vi "FlatToRichnixnet_grpc_ReadStateValue.vi"(5 "OutputClusterType":T1, 11 "InputCluster":T2) -> (3 "OutputCluster":T1)   [LabVIEW 2025, in "grpc-xnet_client.lvlib"]
uses:
  grpc-xnet_client.lvlib
  nixnet_grpc_ReadStateValue_Flat.ctl
  nixnet_grpc_CanCommResponse_Flat.ctl
  nixnet_grpc_CanCommState.ctl
  nixnet_grpc_CanLastErr.ctl
  nixnet_grpc_FlexRayCommResponse_Flat.ctl
  nixnet_grpc_FlexRayPocState.ctl
  nixnet_grpc_FlexRayStats_Flat.ctl
  nixnet_grpc_LinCommResponse_Flat.ctl
  nixnet_grpc_LinCommState.ctl
  nixnet_grpc_SessionInfoResponse_Flat.ctl
  nixnet_grpc_SessionInfoState.ctl
  nixnet_grpc_J1939CommState_Flat.ctl
  nixnet_grpc_TimeLocalNetwork_Flat.ctl
  nixnet_grpc_ReadStateValue.ctl
  nixnet_grpc_ReadStateValue_value/nixnet_grpc_ReadStateValue_value.lvclass
  nixnet_grpc_ReadStateValue_value/nixnet_grpc_ReadStateValue_value.lvclass/nixnet_grpc_ReadStateValue_value.ctl
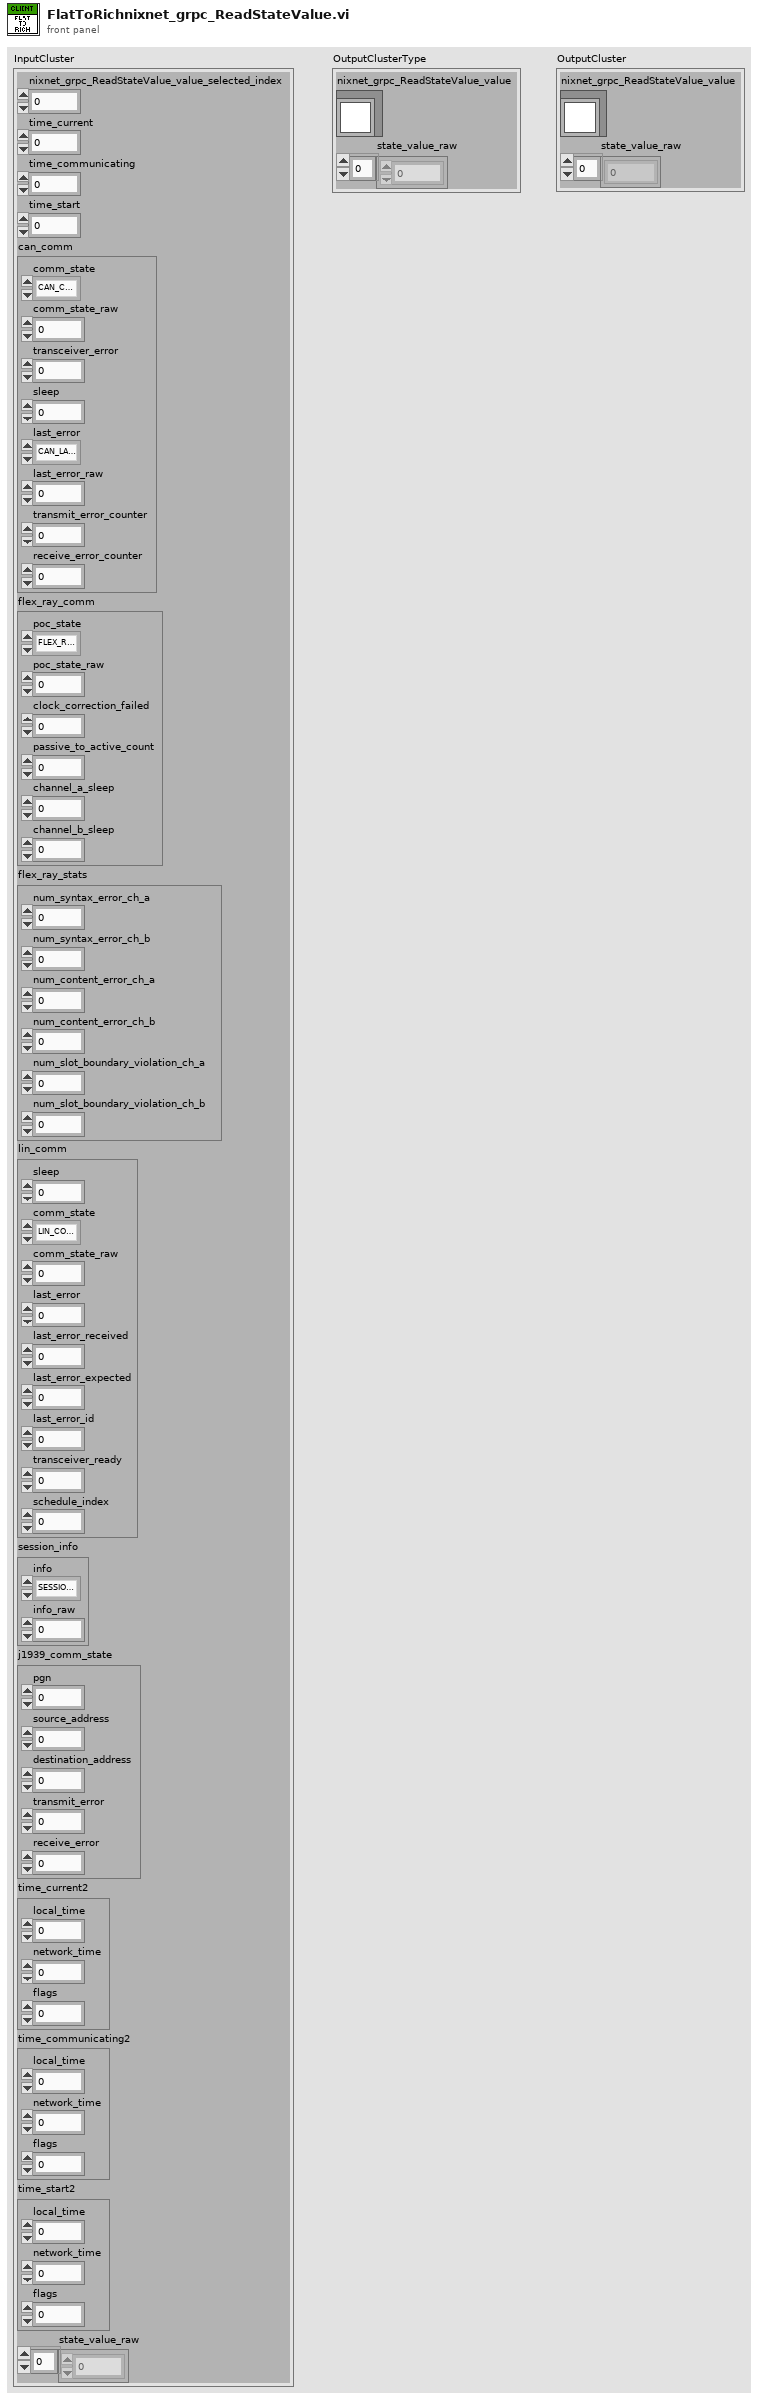
[diagram p1: front panel]
types:
  T1 = typedef "grpc-xnet_client.lvlib/nixnet_grpc_ReadStateValue.ctl" = cluster{"nixnet_grpc_ReadStateValue_value":refnum<class "nixnet_grpc_ReadStateValue_value.lvclass">, "state_value_raw":u8[]}
  T2 = typedef "grpc-xnet_client.lvlib/nixnet_grpc_ReadStateValue_Flat.ctl" = cluster{"nixnet_grpc_ReadStateValue_value_selected_index":i32, "time_current":u64, "time_communicating":u64, "time_start":u64, "can_comm":T3, "flex_ray_comm":T6, "flex_ray_stats":T8, "lin_comm":T9, "session_info":T11, "j1939_comm_state":T13, "time_current2":T14, "time_communicating2":T14, "time_start2":T14, "state_value_raw":u8[]}
  T3 = typedef "grpc-xnet_client.lvlib/nixnet_grpc_CanCommResponse_Flat.ctl" = cluster{"comm_state":T4, "comm_state_raw":u32, "transceiver_error":u32, "sleep":u32, "last_error":T5, "last_error_raw":u32, "transmit_error_counter":u32, "receive_error_counter":u32}
  T4 = typedef "grpc-xnet_client.lvlib/nixnet_grpc_CanCommState.ctl" = enum32{"CAN_COMM_STATE_ERROR_ACTIVE", "CAN_COMM_STATE_ERROR_PASSIVE", "CAN_COMM_STATE_BUS_OFF", "CAN_COMM_STATE_INIT"}
  T5 = typedef "grpc-xnet_client.lvlib/nixnet_grpc_CanLastErr.ctl" = enum32{"CAN_LAST_ERR_NONE", "CAN_LAST_ERR_STUFF", "CAN_LAST_ERR_FORM", "CAN_LAST_ERR_ACK", "CAN_LAST_ERR_BIT_1", "CAN_LAST_ERR_BIT_0", "CAN_LAST_ERR_CRC"}
  T6 = typedef "grpc-xnet_client.lvlib/nixnet_grpc_FlexRayCommResponse_Flat.ctl" = cluster{"poc_state":T7, "poc_state_raw":u32, "clock_correction_failed":u32, "passive_to_active_count":u32, "channel_a_sleep":u32, "channel_b_sleep":u32}
  T7 = typedef "grpc-xnet_client.lvlib/nixnet_grpc_FlexRayPocState.ctl" = enum32{"FLEX_RAY_POC_STATE_DEFAULT_CONFIG", "FLEX_RAY_POC_STATE_READY", "FLEX_RAY_POC_STATE_NORMAL_ACTIVE", "FLEX_RAY_POC_STATE_NORMAL_PASSIVE", "FLEX_RAY_POC_STATE_HALT", "FLEX_RAY_POC_STATE_MONITOR", "FLEX_RAY_POC_STATE_CONFIG"}
  T8 = typedef "grpc-xnet_client.lvlib/nixnet_grpc_FlexRayStats_Flat.ctl" = cluster{"num_syntax_error_ch_a":u32, "num_syntax_error_ch_b":u32, "num_content_error_ch_a":u32, "num_content_error_ch_b":u32, "num_slot_boundary_violation_ch_a":u32, "num_slot_boundary_violation_ch_b":u32}
  T9 = typedef "grpc-xnet_client.lvlib/nixnet_grpc_LinCommResponse_Flat.ctl" = cluster{"sleep":u32, "comm_state":T10, "comm_state_raw":u32, "last_error":u32, "last_error_received":u32, "last_error_expected":u32, "last_error_id":u32, "transceiver_ready":u32, "schedule_index":u32}
  T10 = typedef "grpc-xnet_client.lvlib/nixnet_grpc_LinCommState.ctl" = enum32{"LIN_COMM_STATE_IDLE", "LIN_COMM_STATE_ACTIVE", "LIN_COMM_STATE_INACTIVE"}
  T11 = typedef "grpc-xnet_client.lvlib/nixnet_grpc_SessionInfoResponse_Flat.ctl" = cluster{"info":T12, "info_raw":u32}
  T12 = typedef "grpc-xnet_client.lvlib/nixnet_grpc_SessionInfoState.ctl" = enum32{"SESSION_INFO_STATE_STOPPED", "SESSION_INFO_STATE_STARTED", "SESSION_INFO_STATE_MIX"}
  T13 = typedef "grpc-xnet_client.lvlib/nixnet_grpc_J1939CommState_Flat.ctl" = cluster{"pgn":u32, "source_address":u32, "destination_address":u32, "transmit_error":u32, "receive_error":u32}
  T14 = typedef "grpc-xnet_client.lvlib/nixnet_grpc_TimeLocalNetwork_Flat.ctl" = cluster{"local_time":u64, "network_time":u64, "flags":u32}
  T15 = typedef "grpc-xnet_client.lvlib/nixnet_grpc_CanCommResponse.ctl" = cluster{"comm_state":T4, "comm_state_raw":u32, "transceiver_error":u32, "sleep":u32, "last_error":T5, "last_error_raw":u32, "transmit_error_counter":u32, "receive_error_counter":u32}
  T16 = typedef "grpc-xnet_client.lvlib/nixnet_grpc_FlexRayCommResponse.ctl" = cluster{"poc_state":T7, "poc_state_raw":u32, "clock_correction_failed":u32, "passive_to_active_count":u32, "channel_a_sleep":u32, "channel_b_sleep":u32}
  T17 = typedef "grpc-xnet_client.lvlib/nixnet_grpc_FlexRayStats.ctl" = cluster{"num_syntax_error_ch_a":u32, "num_syntax_error_ch_b":u32, "num_content_error_ch_a":u32, "num_content_error_ch_b":u32, "num_slot_boundary_violation_ch_a":u32, "num_slot_boundary_violation_ch_b":u32}
  T18 = typedef "grpc-xnet_client.lvlib/nixnet_grpc_LinCommResponse.ctl" = cluster{"sleep":u32, "comm_state":T10, "comm_state_raw":u32, "last_error":u32, "last_error_received":u32, "last_error_expected":u32, "last_error_id":u32, "transceiver_ready":u32, "schedule_index":u32}
  T19 = typedef "grpc-xnet_client.lvlib/nixnet_grpc_SessionInfoResponse.ctl" = cluster{"info":T12, "info_raw":u32}
  T20 = typedef "grpc-xnet_client.lvlib/nixnet_grpc_J1939CommState.ctl" = cluster{"pgn":u32, "source_address":u32, "destination_address":u32, "transmit_error":u32, "receive_error":u32}
  T21 = typedef "grpc-xnet_client.lvlib/nixnet_grpc_TimeLocalNetwork.ctl" = cluster{"local_time":u64, "network_time":u64, "flags":u32}
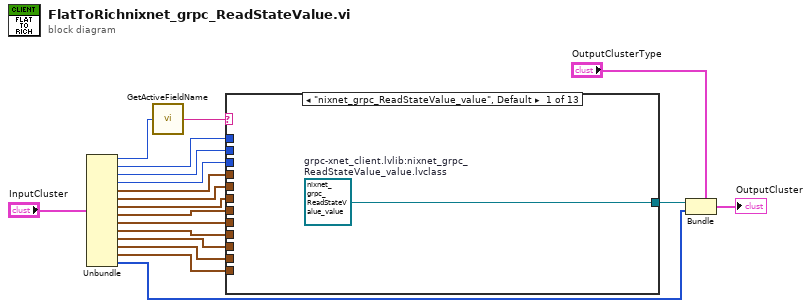
[diagram p0: block diagram]
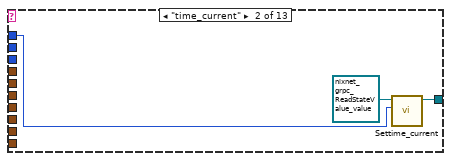
[diagram p2: hidden frame]
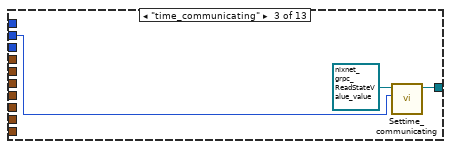
[diagram p3: hidden frame]
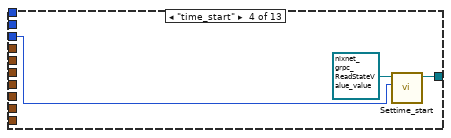
[diagram p4: hidden frame]
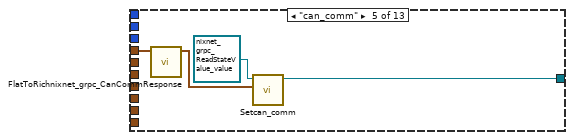
[diagram p5: hidden frame]
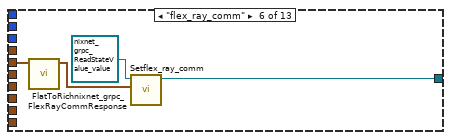
[diagram p6: hidden frame]
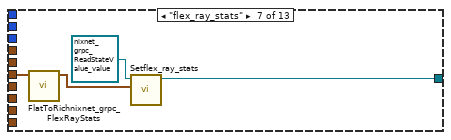
[diagram p7: hidden frame]
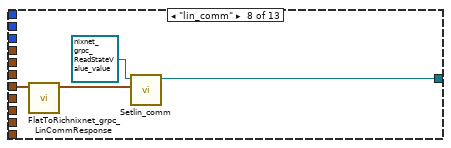
[diagram p8: hidden frame]
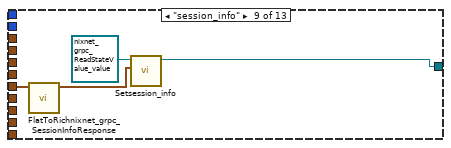
[diagram p9: hidden frame]
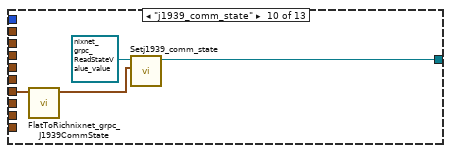
[diagram p10: hidden frame]
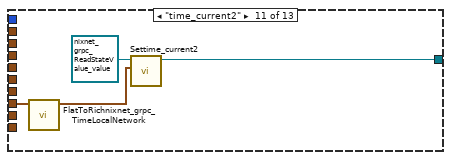
[diagram p11: hidden frame]
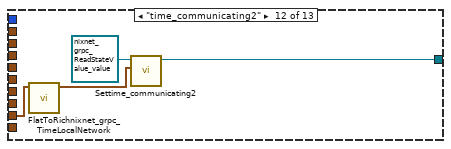
[diagram p12: hidden frame]
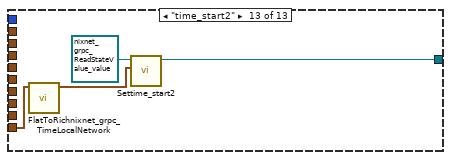
[diagram p13: hidden frame]
diagram:
  n1 = Unbundle "Unbundle"("InputCluster") -> ("nixnet_grpc_ReadStateValue_value_selected_index"=w16:i32, "time_current"=w13:u64, "time_communicating"=w12:u64, "time_start"=w11:u64, "can_comm"=w10:T3, "flex_ray_comm"=w9:T6, "flex_ray_stats"=w8:T8, "lin_comm"=w7:T9, "session_info"=w6:T11, "j1939_comm_state"=w5:T13, "time_current2"=w4:T14, "time_communicating2"=w3:T14, "time_start2"=w2:T14, "state_value_raw"=w1:u8[])
  n2 = call "GetActiveFieldName.vi"("protobuf index"=w16) -> ("oneof field name"=w15:string)
  n3 = case "nixnet_grpc_ReadStateValue_value" shown="\"nixnet_grpc_ReadStateValue_value\", Default" w15 {
    tunnel: [w20 w22 w25 w28 w31 w35 w39 w43 w47 w51 w55 w59 w63] -> w14
    tunnel: w13 -> [_ w23 _ _ _ _ _ _ _ _ _ _ _]
    tunnel: w12 -> [_ _ w26 _ _ _ _ _ _ _ _ _ _]
    tunnel: w11 -> [_ _ _ w29 _ _ _ _ _ _ _ _ _]
    tunnel: w10 -> [_ _ _ _ w33 _ _ _ _ _ _ _ _]
    tunnel: w9 -> [_ _ _ _ _ w37 _ _ _ _ _ _ _]
    tunnel: w8 -> [_ _ _ _ _ _ w41 _ _ _ _ _ _]
    tunnel: w7 -> [_ _ _ _ _ _ _ w45 _ _ _ _ _]
    tunnel: w6 -> [_ _ _ _ _ _ _ _ w49 _ _ _ _]
    tunnel: w5 -> [_ _ _ _ _ _ _ _ _ w53 _ _ _]
    tunnel: w4 -> [_ _ _ _ _ _ _ _ _ _ w57 _ _]
    tunnel: w3 -> [_ _ _ _ _ _ _ _ _ _ _ w61 _]
    tunnel: w2 -> [_ _ _ _ _ _ _ _ _ _ _ _ w65]
    frame "nixnet_grpc_ReadStateValue_value", Default {
      w20 = refnum<class "nixnet_grpc_ReadStateValue_value.lvclass"> refnum  # grpc-xnet_client.lvlib:nixnet_grpc_ReadStateValue_value.lvclass
    }
    frame "time_current" {
      n4 = call "Settime_current.vi"("Set_Val"=w23, "OneOfTemplate in"=refnum<class "nixnet_grpc_ReadStateValue_value.lvclass"> refnum) -> ("OneOfTemplate out"=w22:refnum<class "nixnet_grpc_ReadStateValue_value.lvclass">)  [unwired: 8 in, 1 out]
    }
    frame "time_communicating" {
      n5 = call "Settime_communicating.vi"("Set_Val"=w26, "OneOfTemplate in"=refnum<class "nixnet_grpc_ReadStateValue_value.lvclass"> refnum) -> ("OneOfTemplate out"=w25:refnum<class "nixnet_grpc_ReadStateValue_value.lvclass">)  [unwired: 8 in, 1 out]
    }
    frame "time_start" {
      n6 = call "Settime_start.vi"("Set_Val"=w29, "OneOfTemplate in"=refnum<class "nixnet_grpc_ReadStateValue_value.lvclass"> refnum) -> ("OneOfTemplate out"=w28:refnum<class "nixnet_grpc_ReadStateValue_value.lvclass">)  [unwired: 8 in, 1 out]
    }
    frame "can_comm" {
      n7 = call "FlatToRichnixnet_grpc_CanCommResponse.vi"("InputCluster"=w33) -> ("OutputCluster"=w32:T15)  [unwired: 10 in]
      n8 = call "Setcan_comm.vi"("Set_Val"=w32, "OneOfTemplate in"=refnum<class "nixnet_grpc_ReadStateValue_value.lvclass"> refnum) -> ("OneOfTemplate out"=w31:refnum<class "nixnet_grpc_ReadStateValue_value.lvclass">)  [unwired: 8 in, 1 out]
    }
    frame "flex_ray_comm" {
      n9 = call "FlatToRichnixnet_grpc_FlexRayCommResponse.vi"("InputCluster"=w37) -> ("OutputCluster"=w36:T16)  [unwired: 10 in]
      n10 = call "Setflex_ray_comm.vi"("Set_Val"=w36, "OneOfTemplate in"=refnum<class "nixnet_grpc_ReadStateValue_value.lvclass"> refnum) -> ("OneOfTemplate out"=w35:refnum<class "nixnet_grpc_ReadStateValue_value.lvclass">)  [unwired: 8 in, 1 out]
    }
    frame "flex_ray_stats" {
      n11 = call "FlatToRichnixnet_grpc_FlexRayStats.vi"("InputCluster"=w41) -> ("OutputCluster"=w40:T17)  [unwired: 10 in]
      n12 = call "Setflex_ray_stats.vi"("Set_Val"=w40, "OneOfTemplate in"=refnum<class "nixnet_grpc_ReadStateValue_value.lvclass"> refnum) -> ("OneOfTemplate out"=w39:refnum<class "nixnet_grpc_ReadStateValue_value.lvclass">)  [unwired: 8 in, 1 out]
    }
    frame "lin_comm" {
      n13 = call "FlatToRichnixnet_grpc_LinCommResponse.vi"("InputCluster"=w45) -> ("OutputCluster"=w44:T18)  [unwired: 10 in]
      n14 = call "Setlin_comm.vi"("Set_Val"=w44, "OneOfTemplate in"=refnum<class "nixnet_grpc_ReadStateValue_value.lvclass"> refnum) -> ("OneOfTemplate out"=w43:refnum<class "nixnet_grpc_ReadStateValue_value.lvclass">)  [unwired: 8 in, 1 out]
    }
    frame "session_info" {
      n15 = call "FlatToRichnixnet_grpc_SessionInfoResponse.vi"("InputCluster"=w49) -> ("OutputCluster"=w48:T19)  [unwired: 10 in]
      n16 = call "Setsession_info.vi"("Set_Val"=w48, "OneOfTemplate in"=refnum<class "nixnet_grpc_ReadStateValue_value.lvclass"> refnum) -> ("OneOfTemplate out"=w47:refnum<class "nixnet_grpc_ReadStateValue_value.lvclass">)  [unwired: 8 in, 1 out]
    }
    frame "j1939_comm_state" {
      n17 = call "FlatToRichnixnet_grpc_J1939CommState.vi"("InputCluster"=w53) -> ("OutputCluster"=w52:T20)  [unwired: 10 in]
      n18 = call "Setj1939_comm_state.vi"("Set_Val"=w52, "OneOfTemplate in"=refnum<class "nixnet_grpc_ReadStateValue_value.lvclass"> refnum) -> ("OneOfTemplate out"=w51:refnum<class "nixnet_grpc_ReadStateValue_value.lvclass">)  [unwired: 8 in, 1 out]
    }
    frame "time_current2" {
      n19 = call "FlatToRichnixnet_grpc_TimeLocalNetwork.vi"("InputCluster"=w57) -> ("OutputCluster"=w56:T21)  [unwired: 10 in]
      n20 = call "Settime_current2.vi"("Set_Val"=w56, "OneOfTemplate in"=refnum<class "nixnet_grpc_ReadStateValue_value.lvclass"> refnum) -> ("OneOfTemplate out"=w55:refnum<class "nixnet_grpc_ReadStateValue_value.lvclass">)  [unwired: 8 in, 1 out]
    }
    frame "time_communicating2" {
      n21 = call "FlatToRichnixnet_grpc_TimeLocalNetwork.vi"("InputCluster"=w61) -> ("OutputCluster"=w60:T21)  [unwired: 10 in]
      n22 = call "Settime_communicating2.vi"("Set_Val"=w60, "OneOfTemplate in"=refnum<class "nixnet_grpc_ReadStateValue_value.lvclass"> refnum) -> ("OneOfTemplate out"=w59:refnum<class "nixnet_grpc_ReadStateValue_value.lvclass">)  [unwired: 8 in, 1 out]
    }
    frame "time_start2" {
      n23 = call "FlatToRichnixnet_grpc_TimeLocalNetwork.vi"("InputCluster"=w65) -> ("OutputCluster"=w64:T21)  [unwired: 10 in]
      n24 = call "Settime_start2.vi"("Set_Val"=w64, "OneOfTemplate in"=refnum<class "nixnet_grpc_ReadStateValue_value.lvclass"> refnum) -> ("OneOfTemplate out"=w63:refnum<class "nixnet_grpc_ReadStateValue_value.lvclass">)  [unwired: 8 in, 1 out]
    }
  }
  n25 = Bundle "Bundle"(cluster="OutputClusterType", "nixnet_grpc_ReadStateValue_value"=w14, "state_value_raw"=w1) -> (→"OutputCluster":T1)
